vi "Demo with FGV.vi"() -> ()   [LabVIEW 2014]
uses:
  Power Availabilty Requests/Type Defs/Power Request Type.ctl
  Power Availabilty Requests/Type Defs/Power Availiability Requests Functions.ctl
  Power Requests.lvlib
panel:
  in  "stop":bool
  in  "Keep Screen On":bool
  # "This will prevent the system from \nsleeping when run and will prevent \nthe screen-saver from turing on\nwhen the mouse is hovered over\nthe 'Keep Screen On' button."
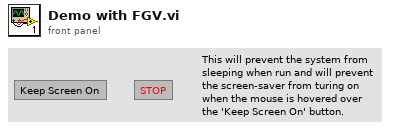
[diagram p1: front panel]
types:
  T1 = typedef "Power Requests.lvlib/Power Availiability Requests Functions.ctl" = enum32{"Power Create Request", "Power Set Request", "Power Clear Request", "Close Handle"}
  T2 = typedef "Power Requests.lvlib/Power Request Type.ctl" = enum32{"Power Request Display Required", "Power Request System Required", "Power Request Away Mode Required", "Power Request Execution Required"}
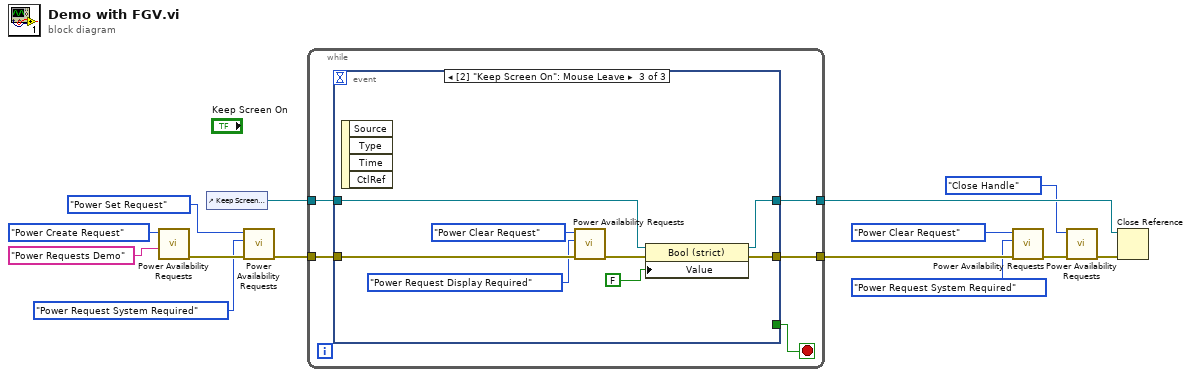
[diagram p0: block diagram]
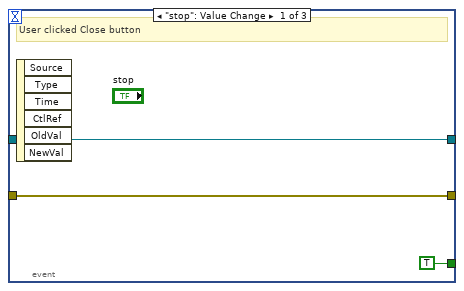
[diagram p2: hidden frame]
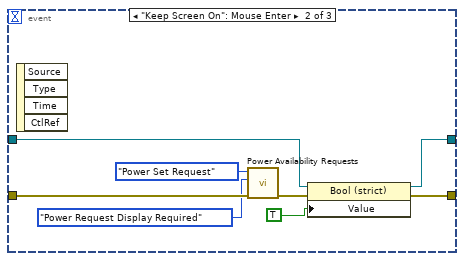
[diagram p3: hidden frame]
diagram:
  n1 = call "Power Availability Requests.vi"("Simple Reason String"="Power Requests Demo", "Power Availability Requests Functions"=Power_Availiability_Requests_Functions."Power Create Request") -> ("error out"=w10:errorcluster)  [unwired: 8 in, 1 out]
  n2 = control-ref of="Keep Screen On"() -> (w14:refnum<vi>)
  n3 = call "Power Availability Requests.vi"("error in (no error)"=w10, "Power Request Type"=Power_Request_Type."Power Request System Required", "Power Availability Requests Functions"=Power_Availiability_Requests_Functions."Power Set Request") -> ("error out"=w9:errorcluster)  [unwired: 7 in, 1 out]
  n4 = while {
    tunnel: w9 -> [w18]
    tunnel: [w17] -> w6
    tunnel: w14 -> [w16]
    tunnel: [w15] -> w13
    stop <- w19 stop-if-true
    n5 = event shown="[2] \"Keep Screen On\": Mouse Leave" {
      selector: _ -> [_ _ _]
      dyn-events: _ -> [_ _ _]
      timeout: _ -> [_ _ _]
      tunnel: [TRUE _ _] -> w19
      tunnel: w18 -> [w22 w26 w34]
      tunnel: [w22 w30 w38] -> w17
      tunnel: w16 -> [w21 w29 w37]
      tunnel: [w21 w28 w36] -> w15
      event "stop": Value Change {
        # "User clicked Close button"
        n6 = event-data() -> ()  [unwired: 1 in, 6 out]
      }
      event "Keep Screen On": Mouse Enter {
        n7 = event-data() -> ()  [unwired: 1 in, 4 out]
        n8 = call "Power Availability Requests.vi"("error in (no error)"=w26, "Power Request Type"=Power_Request_Type."Power Request Display Required", "Power Availability Requests Functions"=Power_Availiability_Requests_Functions."Power Set Request") -> ("error out"=w24:errorcluster)  [unwired: 7 in, 1 out]
        n9 = property class="Bool (strict)"(reference=w29, error in=w24, "Value"=TRUE) -> (reference out=w28:refnum<vi>, error out=w30:errorcluster)
      }
      event "Keep Screen On": Mouse Leave {
        n10 = event-data() -> ()  [unwired: 1 in, 4 out]
        n11 = call "Power Availability Requests.vi"("error in (no error)"=w34, "Power Request Type"=Power_Request_Type."Power Request Display Required", "Power Availability Requests Functions"=Power_Availiability_Requests_Functions."Power Clear Request") -> ("error out"=w33:errorcluster)  [unwired: 7 in, 1 out]
        n12 = property class="Bool (strict)"(reference=w37, error in=w33, "Value"=FALSE) -> (reference out=w36:refnum<vi>, error out=w38:errorcluster)
      }
    }
  }
  n13 = call "Power Availability Requests.vi"("error in (no error)"=w6, "Power Request Type"=Power_Request_Type."Power Request System Required", "Power Availability Requests Functions"=Power_Availiability_Requests_Functions."Power Clear Request") -> ("error out"=w4:errorcluster)  [unwired: 7 in, 1 out]
  n14 = call "Power Availability Requests.vi"("error in (no error)"=w4, "Power Availability Requests Functions"=Power_Availiability_Requests_Functions."Close Handle") -> ("error out"=w3:errorcluster)  [unwired: 8 in, 1 out]
  n15 = Close Reference(reference=w13, error in (no error)=w3) -> ()  [unwired: 1 out]
